vi "Configure 2Wire Resistance.vi"(0 "VISA resource name":refnum<visa-resource-name>, 1 "NPLC":u16(ring) items=["0.00005", "1", "12", "15"], 5 "Auto Range? (T: Auto)":bool, 7 "Manual Range":dbl, 9 "Aperture Seconds":dbl, 11 "error in (no error)":errorcluster) -> (4 "VISA resource name out":refnum<visa-resource-name>, 15 "error out":errorcluster)   [LabVIEW 2009, in "Keithley DMM7510.lvlib"]
doc: "This VI configures the 2 wire Resistance."
uses:
  Keithley DMM7510.lvlib
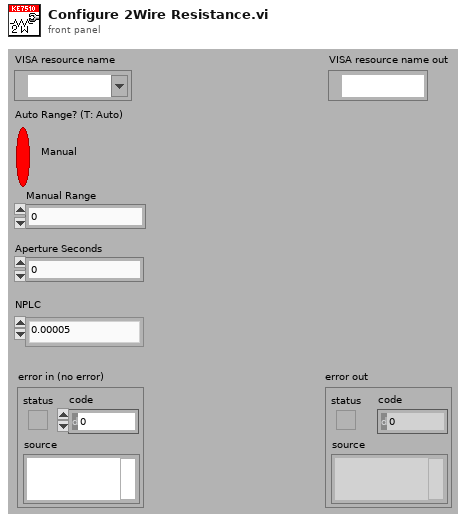
[diagram p1: front panel]
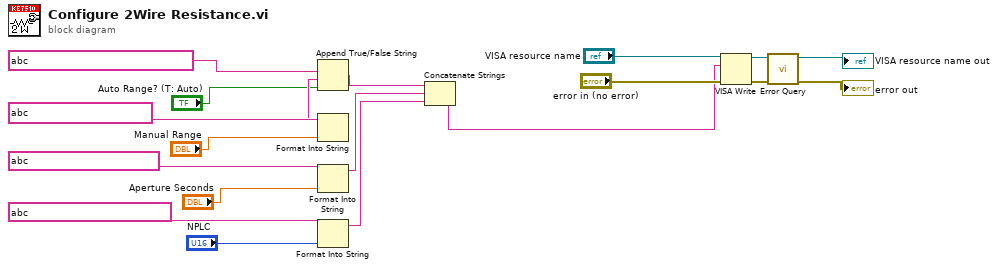
[diagram p0: block diagram]
diagram:
  n1 = Format Into String(format string=string ?, "Manual Range") -> (resulting string=w11:string)  [unwired: 2 in, 1 out]
  n2 = Append True/False String(1:"Auto Range? (T: Auto)", 2:w11, 3:string ?) -> (0:w8:string)  [unwired: 1 in]
  n3 = Format Into String(format string=string ?, "Aperture Seconds") -> (resulting string=w7:string)  [unwired: 2 in, 1 out]
  n4 = Format Into String(format string=string ?, "NPLC") -> (resulting string=w6:string)  [unwired: 2 in, 1 out]
  n5 = Concatenate Strings(w8, w7, w6) -> (w5:string)
  n6 = VISA Write(VISA resource name="VISA resource name", write buffer=w5, error in (no error)="error in (no error)") -> (VISA resource name out=w19:refnum<visa-resource-name>, error out=w18:errorcluster)  [unwired: 1 out]
  n7 = call "Error Query.vi"("error in (no error)"=w18, "VISA resource name"=w19) -> ("error out"=→"error out":errorcluster, "VISA resource name out"=→"VISA resource name out":refnum<visa-resource-name>)  [unwired: 6 in, 2 out]
